vi "PCO_GetHWIOSignalCount.vi"(8 "error in (no error)":errorcluster {"code" format="%x"}, 11 "ph":u64) -> (0 "error out":errorcluster {"code" format="%x"}, 1 "wNumSignals":u16, 2 "ErrorMessage":i32 format="%x", 3 "ph out":u64)   [LabVIEW 2019, in "SDK.lvlib" / "TimingControl.lvlib"]
doc: "<b>Description:</b>\nThis function returns the number of hardware I/O signal lines, which are available at the camera.\nFunction PCO_GetHWIOSignalDescriptor must be called to get a description of the available options for a distinct I/O signal line. With this information the current settings can be changed with PCO_SetHWIOSignal and queried with PCO_GetHWIOSignal.\n\n<b>Supported camera type:</b>\npco.edge, pco.dimax\n\n<b>Descriptor dependency:</b>\ndwGeneralCapsDESC1: HW_IO_SIGNAL_DESCRIPTOR"
uses:
  TimingControl.lvlib
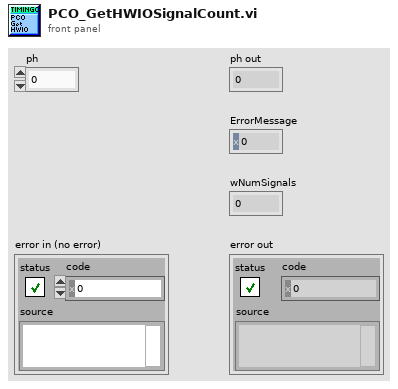
[diagram p1: front panel]
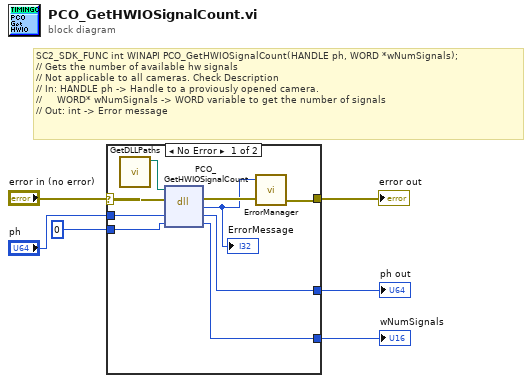
[diagram p0: block diagram]
diagram:
  # "SC2_SDK_FUNC int WINAPI PCO_GetHWIOSignalCount(HANDLE ph, WORD *wNumSignals);\n// Gets the number of available hw signals\n// Not applicable to all cameras. Check Description\n// In: HANDLE ph -> Handle to a proviously opened camera.\n//     WORD* wNumSignals -> WORD variable to get the number of signals\n// Out: int -> Error message"
  n1 = case shown="No Error" "error in (no error)" {
    selector: "error in (no error)" -> [w8 w18]
    tunnel: "ph" -> [w15 w17]
    tunnel: [w14 w17] -> w5
    tunnel: u16 0 ("wNumSignals") -> [w13 w16]
    tunnel: [w12 w16] -> w3
    tunnel: [w10 w18] -> w2
    frame No Error {
      n2 = call "GetDLLPaths.vi"() -> ("SC2_Cam_Path"=w7:path)  [unwired: 9 in, 2 out]
      n3 = dll-call lib="?" fn="PCO_GetHWIOSignalCount"(path in=w7, error in=w8, "ph"=w15, "wNumSignals"=w13) -> (error out=w11:errorcluster, "return type"=w9:i32, "ph"=w14:u64, "wNumSignals"=w12:u16)  [unwired: 1 in, 1 out]
      "ErrorMessage" <- w9
      n4 = call "ErrorManager.vi"("error in (no error)"=w11, "error code"=w9) -> ("error out"=w10:errorcluster)  [unwired: 3 in]
    }
    frame Error {
    }
  }
  "ph out" <- w5
  "wNumSignals" <- w3
  "error out" <- w2
